vi "Array Exponential Dampening.vi"(8 "Error In":errorcluster, 9 "Damping Factor (default: 2)":dbl=2.0, 11 "Array":dbl[](array[numeric])) -> (0 "Error Out":errorcluster, 3 "Dampened Array":dbl[](array[numeric]))   [LabVIEW 2021, in "Arrays.lvlib"]
doc: "Multiplies an <B>Array</B> by exp(-K*i/n) where K is the <b>Damping Factor</b>, i the element index and n the number of elements in the array."
uses:
  Arrays.lvlib
panel:
  # "see the AlliGator License on the block diagram (Ctrl+E or Window:Show Block Diagram)"
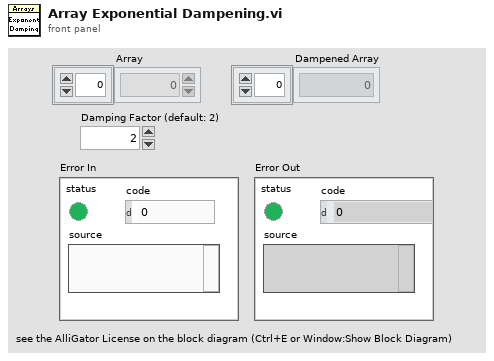
[diagram p1: front panel]
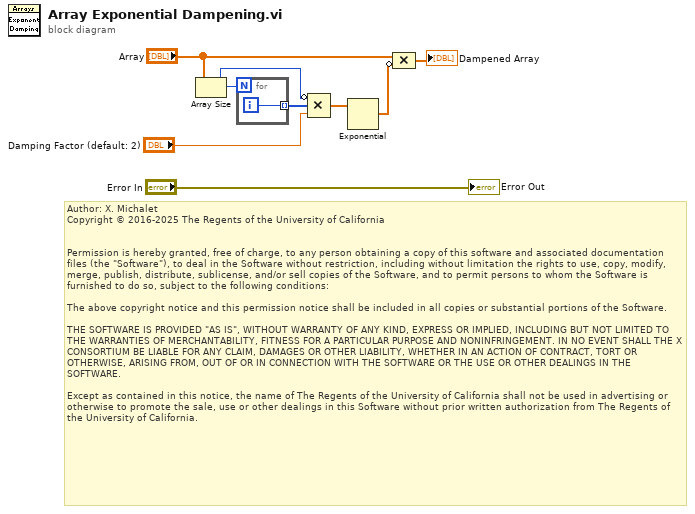
[diagram p0: block diagram]
diagram:
  # "Author: X. Michalet\nCopyright © 2016-2025 The Regents of the University of California\n \n\nPermission is hereby granted, free of charge, to any person obtaining a copy of this software and associated documentation files (the \"Software\"), to deal in the Software without restriction, including without limitation the rights to use, copy, modify, merge, publish, distribute, sublicense, and/or sell copies of the Software, and to permit persons to whom the Software is furnished to do so, subject to the following conditions:\n\nThe above copyright notice and this permission notice shall be included in all copies or substantial portions of the Software.\n\nTHE SOFTWARE IS PROVIDED \"AS IS\", WITHOUT WARRANTY OF ANY KIND, EXPRESS OR IMPLIED, INCLUDING BUT NOT LIMITED TO THE WARRANTIES OF MERCHANTABILITY, FITNESS FOR A PARTICULAR PURPOSE AND NONINFRINGEMENT. IN NO EVENT SHALL THE X CONSORTIUM BE LIABLE FOR ANY CLAIM, DAMAGES OR OTHER LIABILITY, WHETHER IN AN ACTION OF CONTRACT, TORT OR OTHERWISE, ARISING FROM, OUT OF OR IN CONNECTION WITH THE SOFTWARE OR THE USE OR OTHER DEALINGS IN THE SOFTWARE.\n\nExcept as contained in this notice, the name of The Regents of the University of California shall not be used in advertising or otherwise to promote the sale, use or other dealings in this Software without prior written authorization from The Regents of the University of California."
  n1 = Array Size(array="Array") -> (size(s)=w5:i32)
  n2 = for {
    N: w5 -> [_]
    tunnel: [w9] -> w7 mode=indexing
    i -> [w9]
  }
  n3 = Compound Arithmetic op=MULTIPLY(invert w5, w7, "Damping Factor (default: 2)") -> (w6:dbl[])
  n4 = Exponential(1:w6) -> (0:w3:dbl[])
  n5 = Compound Arithmetic op=MULTIPLY("Array", invert w3) -> (→"Dampened Array":dbl[])
  "Error Out" <- "Error In"
